vi "Weird Master.vi"() -> ()   [LabVIEW 2012]
uses:
  API/Master/Modbus Master.lvclass
  Master Function Definition/Master Function Definition.lvclass
  Network Protocol/Network Master/TCP/TCP Master.lvclass
  Transmission Data Unit/RTU/RTU Data Unit.lvclass
  Transmission Data Unit/ASCII/ASCII Data Unit.lvclass
  Transmission Data Unit/Serial Interface/Serial Data Unit.lvclass
  Data Model/Identification Parameters.ctl
  Data Model/Device Data Model.lvclass
  Master Function Definition/Read Device ID code.ctl
panel:
  in  "Serial Type":enum16{"RTU", "ASCII"}(ring)
  in  "Unit ID":u8=1
  out "loop time":dbl
  in  "Read Device ID code":T1
  in  "Object ID":u8
  out "Objects":T2[](array[typedef]) {"Object ID" format="%x"}
  out "exception status":u8
  out "discrete inputs":bool[](array[boolean])
  out "Input Registers":u16[](array[numeric])=[0, 0, 2, 2]
  out "error out":errorcluster
  out "Holding Registers":u16[](array[numeric])=[0, 0, 2, 2]
  in  "Write Single Register":u16[](array[numeric])=[0, 0, 2, 2]
  in  "Write Multiple Registers":cluster{"Set Registers":bool, u16[]}={"Set Registers"=FALSE, [0, 0, 2, 2]}
  in  "Write Multiple Coils":T3={"Write Single Coils 2"=[TRUE, FALSE, FALSE, TRUE], "Set Coils"=FALSE}
  in  "Write Single Coils":bool[](array[boolean])=[FALSE, FALSE, FALSE, FALSE] caption="Coils to Write"
  in  "Address":string="localhost"
  in  "Stop":bool
  out "Coils":bool[](array[boolean])=[TRUE, FALSE, FALSE, TRUE] caption="Slave Discrete Inputs"
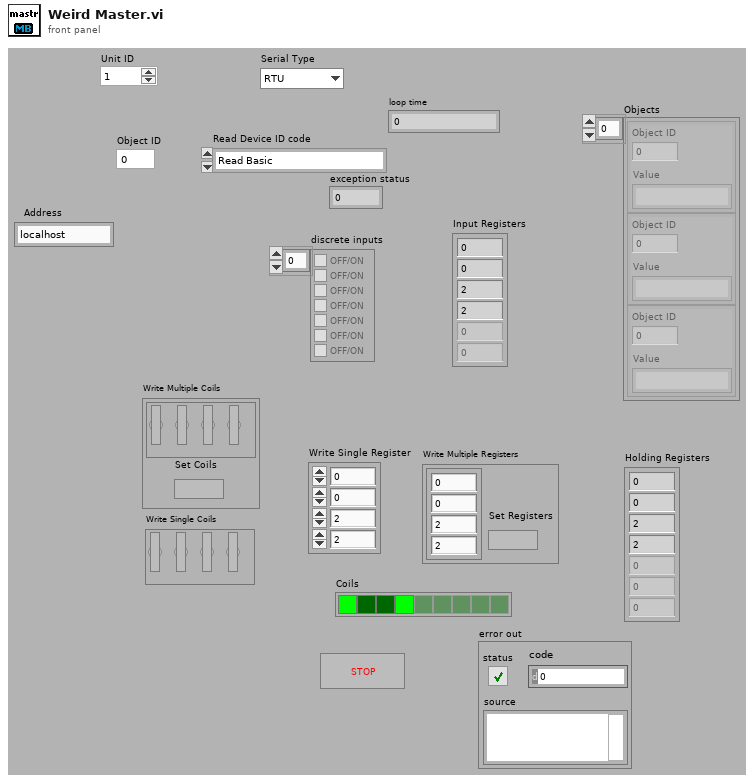
[diagram p1: front panel]
types:
  T1 = typedef "Device Data Model.lvclass/Read Device ID code.ctl" = enum8{"Read Basic", "Read Regular", "Read Extended", "Read Specific"}
  T2 = typedef "Device Data Model.lvclass/Identification Parameters.ctl" = cluster{"Object ID":u8, "Value":string}
  T3 = cluster{"Write Single Coils 2":bool[], "Set Coils":bool}
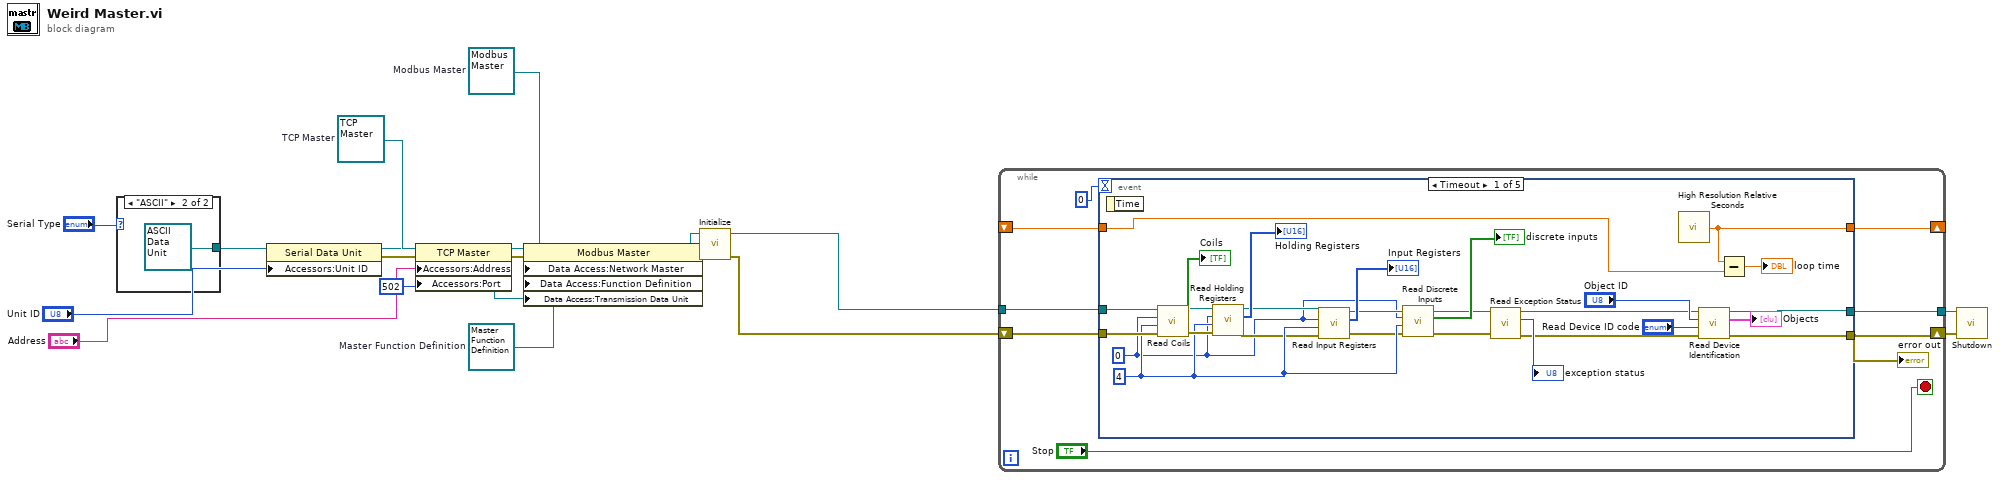
[diagram p0: block diagram]
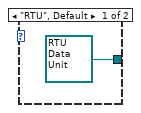
[diagram p2: hidden frame]
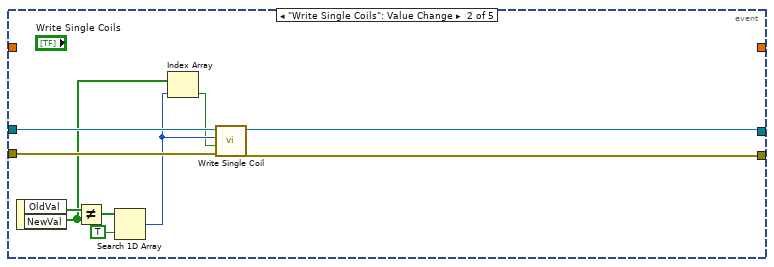
[diagram p3: hidden frame]
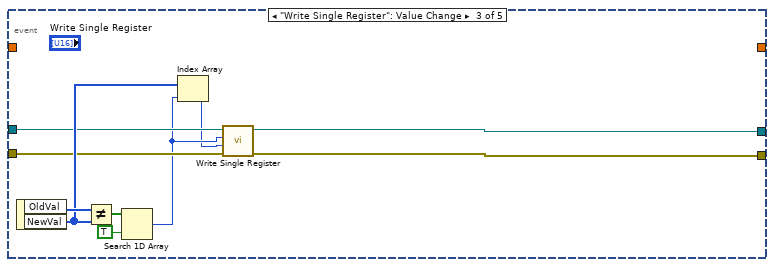
[diagram p4: hidden frame]
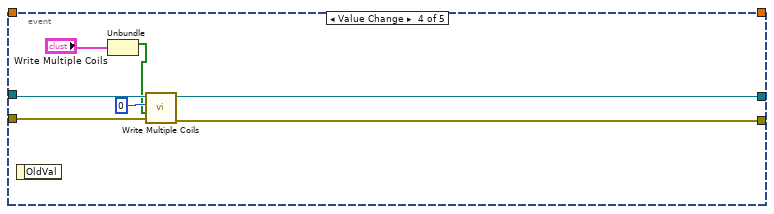
[diagram p5: hidden frame]
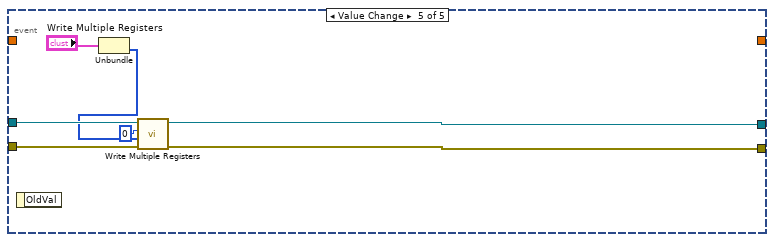
[diagram p6: hidden frame]
diagram:
  w16 = refnum<class "TCP Master.lvclass"> refnum  # TCP Master
  w12 = refnum<class "Master Function Definition.lvclass"> refnum  # Master Function Definition
  w15 = refnum<class "Modbus Master.lvclass"> refnum  # Modbus Master
  n1 = case shown="\"ASCII\"" "Serial Type" {
    tunnel: [refnum<class "RTU Data Unit.lvclass"> refnum ("RTU Data Unit") refnum<class "ASCII Data Unit.lvclass"> refnum ("ASCII Data Unit")] -> w4
    frame "RTU", Default {
    }
    frame "ASCII" {
    }
  }
  n2 = property class="Serial Data Unit"(reference=w4, "Accessors:Unit ID"="Unit ID") -> (reference out=w3:refnum<class "Serial Data Unit.lvclass">, error out=w2:errorcluster)  [unwired: 1 in]
  n3 = property class="TCP Master"(reference=w16, error in=w2, "Accessors:Address"="Address", "Accessors:Port"=u16 502 ("Port")) -> (reference out=w13:refnum<class "TCP Master.lvclass">, error out=w14:errorcluster)
  n4 = property class="Modbus Master"(reference=w15, error in=w14, "Data Access:Network Master"=w13, "Data Access:Function Definition"=w12, "Data Access:Transmission Data Unit"=w3) -> (reference out=w10:refnum<class "Modbus Master.lvclass">, error out=w11:errorcluster)
  n5 = call-dynamic "Initialize.vi"("error in"=w11, "Modbus master in"=w10) -> ("error out"=w8:errorcluster, "Modbus master out"=w9:refnum<class "Modbus Master.lvclass">)  [unwired: 8 in]
  n6 = while {
    tunnel: w9 -> [w25]
    tunnel: [w24] -> w17
    shift-right: [w27] -> w18
    shift-left: w8 -> [w23]
    shift-right: [w22] -> _
    shift-left: _ -> [w21]
    stop <- "Stop" stop-if-true
    n7 = event shown="[0] Timeout" {
      selector: _ -> [_ _ _ _ _]
      dyn-events: _ -> [_ _ _ _ _]
      timeout: 0 -> [_ _ _ _ _]
      tunnel: [w32 w63 w71 w78 w85] -> w27
      tunnel: w25 -> [w55 w65 w69 w81 w87]
      tunnel: [w34 w62 w70 w77 w86] -> w24
      tunnel: w23 -> [w54 w64 w68 w80 w88]
      tunnel: [w31 _ _ _ _] -> w22
      tunnel: w21 -> [w30 _ _ _ _]
      event Timeout {
        w48 = u16 4 ("Number of coils")
        w41 = u16 0 ("Starting Address")
        n8 = event-data() -> ()  [unwired: 2 out]
        n9 = call-dynamic "Read Coils.vi"("error in"=w54, "number of inputs"=w48, "starting address"=w41, "Modbus master in"=w55) -> ("error out"=w51:errorcluster, "coils"=→"Coils":bool[], "Modbus master out"=w52:refnum<class "Modbus Master.lvclass">)  [unwired: 5 in]
        n10 = call-dynamic "Read Holding Registers.vi"("error in"=w51, "number of inputs"=w48, "starting address"=w41, "Modbus master in"=w52) -> ("error out"=w44:errorcluster, "register values"=→"Holding Registers":u16[], "Modbus master out"=w45:refnum<class "Modbus Master.lvclass">)  [unwired: 5 in]
        n11 = call-dynamic "Read Input Registers.vi"("error in"=w44, "number of inputs"=w48, "starting address"=w41, "Modbus master in"=w45) -> ("error out"=w42:errorcluster, "register values"=→"Input Registers":u16[], "Modbus master out"=w43:refnum<class "Modbus Master.lvclass">)  [unwired: 5 in]
        n12 = call-dynamic "Read Discrete Inputs.vi"("error in"=w42, "number of inputs"=w48, "starting address"=w41, "Modbus master in"=w43) -> ("error out"=w39:errorcluster, "discrete inputs"=→"discrete inputs":bool[], "Modbus master out"=w40:refnum<class "Modbus Master.lvclass">)  [unwired: 5 in]
        n13 = call-dynamic "Read Exception Status.vi"("error in"=w39, "Modbus master in"=w40) -> ("error out"=w33:errorcluster, "exception status"=→"exception status":u8, "Modbus master out"=w35:refnum<class "Modbus Master.lvclass">)  [unwired: 7 in]
        n14 = call <vilib>:"High Resolution Relative Seconds.vi"() -> ("relative seconds"=w31:dbl)
        n15 = call-dynamic "Read Device Identification.vi"("error in"=w33, "read device ID code"="Read Device ID code", "object ID"="Object ID", "Modbus master in"=w35) -> ("error out"=w32:errorcluster, "objects"=→"Objects":T2[], "Modbus master out"=w34:refnum<class "Modbus Master.lvclass">)  [unwired: 5 in]
        n16 = Subtract(x=w31, y=w30) -> (x-y=→"loop time":dbl)
      }
      event "Write Single Coils": Value Change {
        n17 = event-data() -> ("OldVal"=w61:bool[], "NewVal"=w58:bool[])  [unwired: 1 out]
        n18 = Not Equal?(x=w61, y=w58) -> (x != y?=w60:bool[])
        n19 = Search 1D Array(1D array=w60, element=TRUE) -> (index of element=w57:i32)  [unwired: 1 in]
        n20 = Index Array(array=w58, index=w57) -> (element=w56:bool)
        n21 = call-dynamic "Write Single Coil.vi"("error in"=w64, "coil to write"=w56, "address"=w57, "Modbus master in"=w65) -> ("error out"=w63:errorcluster, "Modbus master out"=w62:refnum<class "Modbus Master.lvclass">)  [unwired: 6 in]
      }
      event "Write Single Register": Value Change {
        n22 = event-data() -> ("OldVal"=w73:u16[], "NewVal"=w72:u16[])  [unwired: 1 out]
        n23 = Not Equal?(x=w73, y=w72) -> (x != y?=w75:bool[])
        n24 = Search 1D Array(1D array=w75, element=TRUE) -> (index of element=w67:i32)  [unwired: 1 in]
        n25 = Index Array(array=w72, index=w67) -> (element=w66:u16)
        n26 = call-dynamic "Write Single Register.vi"("error in"=w68, "register to write"=w66, "address"=w67, "Modbus master in"=w69) -> ("error out"=w71:errorcluster, "Modbus master out"=w70:refnum<class "Modbus Master.lvclass">)  [unwired: 6 in]
      }
      event "Write Multiple Coils.Set Coils": Value Change {
        n27 = event-data() -> ()  [unwired: 2 out]
        n28 = Unbundle("Write Multiple Coils") -> ("Write Single Coils 2"=w76:bool[])  [unwired: 1 out]
        n29 = call-dynamic "Write Multiple Coils.vi"("error in"=w80, "coils to write"=w76, "starting address"=u16 0 ("Starting Address"), "Modbus master in"=w81) -> ("error out"=w78:errorcluster, "Modbus master out"=w77:refnum<class "Modbus Master.lvclass">)  [unwired: 6 in]
      }
      event "Write Multiple Registers.Set Registers": Value Change {
        n30 = event-data() -> ()  [unwired: 2 out]
        n31 = Unbundle("Write Multiple Registers") -> (w83:u16[])  [unwired: 1 out]
        n32 = call-dynamic "Write Multiple Registers.vi"("error in"=w88, "registers to write"=w83, "starting address"=u16 0 ("Starting Address"), "Modbus master in"=w87) -> ("error out"=w85:errorcluster, "Modbus master out"=w86:refnum<class "Modbus Master.lvclass">)  [unwired: 6 in]
      }
    }
    "error out" <- w27
  }
  n33 = call-dynamic "Shutdown.vi"("error in"=w18, "Modbus master in"=w17) -> ()  [unwired: 9 in, 1 out]
